vi "dfd_Check Real.vi"(1 "complex":cdb format="%.2f") -> (0 "real?":bool)   [LabVIEW 2017, in "NI_DigFilter_Design.lvlib"]
uses:
  <vilib>/addons/Digital Filter Design/NI_DigFilter_Design.lvlib
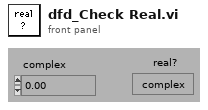
[diagram p1: front panel]
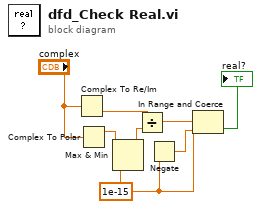
[diagram p0: block diagram]
diagram:
  w3 = 1e-15
  n1 = Complex To Re/Im(x + iy="complex") -> (y=w7:dbl)  [unwired: 1 out]
  n2 = Complex To Polar(r * e^(i*theta)="complex") -> (r=w2:dbl)  [unwired: 1 out]
  n3 = Max & Min(x=w2, y=w3) -> (max(x,y)=w1:dbl)  [unwired: 1 out]
  n4 = Divide(x=w7, y=w1) -> (x/y=w5:dbl)
  n5 = Negate(x=w3) -> (-x=w6:dbl)
  n6 = In Range and Coerce(upper limit=w3, x=w5, lower limit=w6) -> (In Range?=→"real?":bool)  [unwired: 1 out]
